vi "Serial Port Write 2.vi"(8 "string to write":string, 11 "port number":i32) -> (0 "error code":i32, 3 "port number out":i32)   [LabVIEW 2010]
doc: "Writes the data in string to write to the serial port indicated in port number."
uses:
  <vilib>/Instr/serial.llb/serpConfig.vi
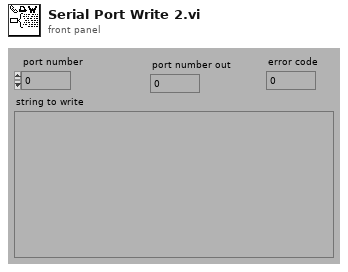
[diagram p1: front panel]
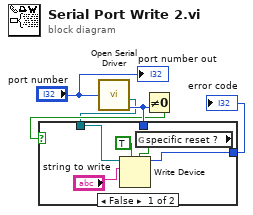
[diagram p0: block diagram]
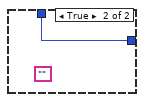
[diagram p2: hidden frame]
diagram:
  n1 = call <vilib>:"Open Serial Driver.vi"("port number"="port number") -> ("output refnum"=w2:refnum<visa-resource-name>, "output error"=w4:i32)  [unwired: 2 out]
  n2 = Not Equal To 0?(x=w4) -> (x != 0?=w3:bool)
  n3 = case shown="False" w3 {
    tunnel: [w8 w11] -> w5
    tunnel: w4 -> [_ w11]
    tunnel: w2 -> [w10 _]
    frame False {
      n4 = global read "serpConfig.vi" "specific reset ?"() -> (w6:bool)
      n5 = Write Device(4:w6, 6:TRUE, 9:"string to write", 10:w10) -> (3:w8:i16)  [unwired: 3 in, 2 out]
    }
    frame True {
      (unwired) ""
    }
  }
  "error code" <- w5
  "port number out" <- "port number"
